vi "Calc_rhozero.vi"(0 "Q":dbl[](array[numeric])) -> (7 "rho+":dbl[](array[numeric]))   [LabVIEW 2018]
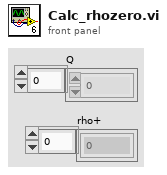
[diagram p1: front panel]
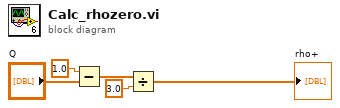
[diagram p0: block diagram]
diagram:
  n1 = Subtract(x=1.0, y="Q") -> (x-y=w2:dbl[])
  n2 = Divide(x=w2, y=3.0) -> (x/y=→"rho+":dbl[])
